vi "Inches to Ticks.vi"(1 "Inches":dbl format="%#_13g") -> (0 "Ticks":dbl format="%#_13g")   [LabVIEW 2016]
panel:
  out "error out":errorcluster
  in  "error in":errorcluster
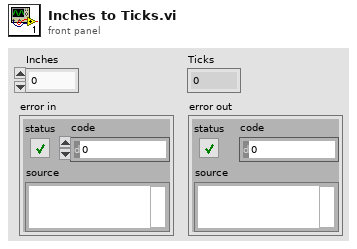
[diagram p1: front panel]
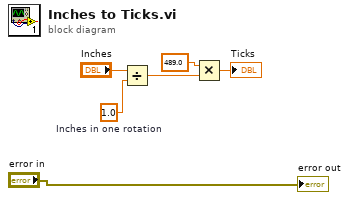
[diagram p0: block diagram]
diagram:
  w3 = 1.0  # Inches in one rotation
  n1 = Divide(x="Inches", y=w3) -> (x/y=w5:dbl)
  n2 = Multiply(x=489.0, y=w5) -> (x*y=→"Ticks":dbl)
  "error out" <- "error in"
